vi "Define_Place_of_Displacement-1.vi"(3 "[IN] Indexes for Jumps":i32[](array[numeric]), 4 "[IN] Subtrack":dbl[](array[numeric]), 5 "[IN] Tracks":dbl[][](array[numeric])) -> (1 "[OUT] Index of \"11\" Dis\nplacement in Subtrack":i32)   [LabVIEW 2013]
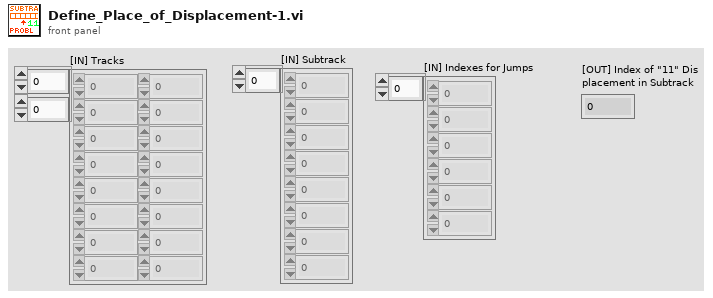
[diagram p1: front panel]
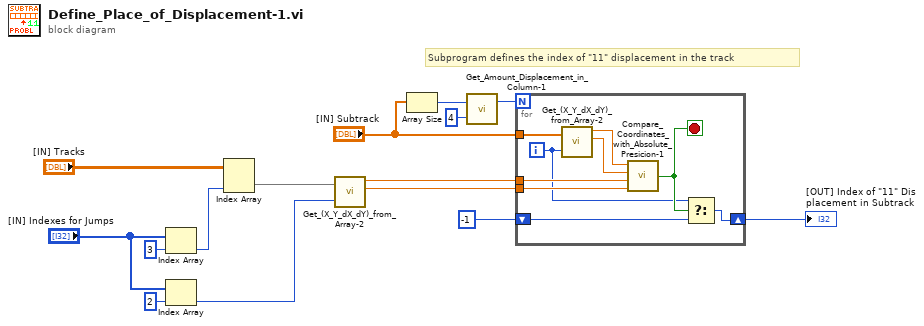
[diagram p0: block diagram]
diagram:
  # "Subprogram defines the index of \"11\" displacement in the track"
  n1 = Index Array(array="[IN] Indexes for Jumps", index=3) -> (element=w13:i32)
  n2 = Index Array(array="[IN] Indexes for Jumps", index=2) -> (element=w9:i32)
  n3 = Index Array(array="[IN] Tracks", index (col)=w13) -> (element=w10:dbl[])  [unwired: 1 in]
  n4 = call "Get_(X_Y_dX_dY)_from_Array-2.vi"("(X,Y,dX,dY)"=w10, "Index of Displacement"=w9) -> ("X"=w4:dbl, "Y"=w3:dbl)  [unwired: 2 out]
  n5 = Array Size(array="[IN] Subtrack") -> (size(s)=w8:i32)
  n6 = call "Get_Amount_Displacement_in_Column-1.vi"("multiplier"=4, "# Rows"=w8) -> ("Displ amount"=w6:i32)  [unwired: 1 out]
  n7 = for {
    N: w6 -> [_]
    tunnel: "[IN] Subtrack" -> [w24]
    tunnel: w4 -> [w21]
    tunnel: w3 -> [w20]
    shift-right: [w17] -> w1
    shift-left: -1 -> [w18]
    i -> [w16]
    stop <- w19 stop-if-true
    n8 = call "Get_(X_Y_dX_dY)_from_Array-2.vi"("(X,Y,dX,dY)"=w24, "Index of Displacement"=w16) -> ("X"=w23:dbl, "Y"=w22:dbl)  [unwired: 2 out]
    n9 = call "Compare_Coordinates_with_Absolute_Presicion-1.vi"("X 1"=w23, "Y 1"=w22, "X 2"=w21, "Y 2"=w20) -> ("[OUT] Same coordinates?"=w19:bool)  [unwired: 1 in]
    n10 = Select(t=w16, s=w19, f=w18) -> (s? t:f=w17:i32)
  }
  "[OUT] Index of \"11\" Dis\nplacement in Subtrack" <- w1
